vi "Get Current Step.vi"(8 "error in (no error)":errorcluster, 11 "Sequencer in":refnum<class "Sequencer.lvclass">) -> (0 "error out":errorcluster, 3 "Current Step":u32)   [LabVIEW 2024, in "Ramses Sequencer.lvlib" / "Sequencer.lvclass"]
uses:
  Sequencer.lvclass
  C:/Program Files (x86)/Enterative/Ramses Framework/Ramses Framework.lvlibp/Service/Service.lvclass
  Program Files (x86)/Enterative/Ramses Framework/Ramses Framework.lvlibp/Service/Service.lvclass
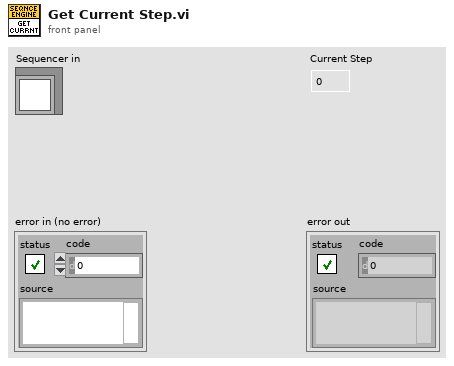
[diagram p1: front panel]
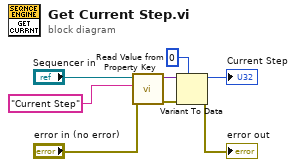
[diagram p0: block diagram]
diagram:
  n1 = call "Read Value from Property Key.vi"("error in (no error)"="error in (no error)", "Key"="Current Step", "Service in"="Sequencer in") -> ("error out"=w2:errorcluster, "Value"=w1:variant)  [unwired: 7 in]
  n2 = Variant To Data(error in=w2, type=u32 0, Variant=w1) -> (data=→"Current Step":u32, error out=→"error out":errorcluster)
